vi "Get date.vi"() -> (0 "date/time string":string)   [LabVIEW 2018]
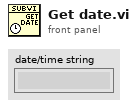
[diagram p1: front panel]
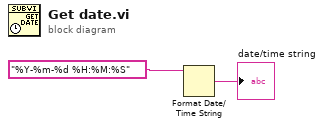
[diagram p0: block diagram]
diagram:
  n1 = Format Date/Time String(time format string (%c)="%Y-%m-%d %H:%M:%S") -> (date/time string=→"date/time string":string)  [unwired: 2 in]
